vi "Flatten Readable.vi"(8 "error in (no error)":errorcluster, 11 "Reader.lvclass":refnum<class "Reader.lvclass">) -> (0 "error out":errorcluster)   [LabVIEW 2009, in "Reader.lvclass"]
uses:
  Reader.lvclass
  Reader.lvclass/Reader.ctl
  Instruments/Utility Classes/Readable/Readable.lvclass
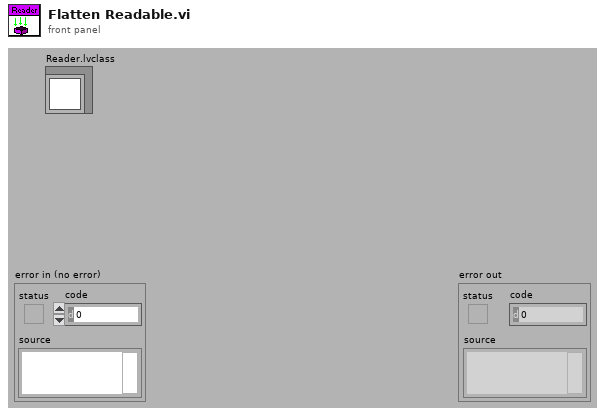
[diagram p1: front panel]
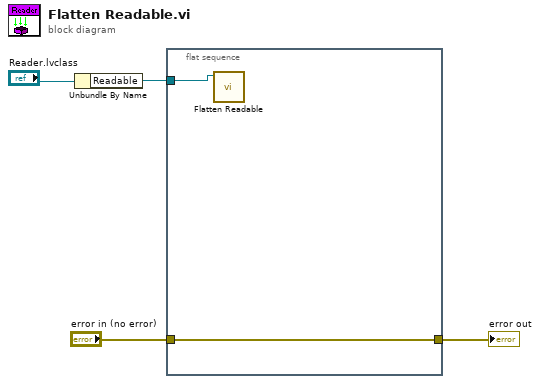
[diagram p0: block diagram]
diagram:
  n1 = Unbundle By Name("Reader.lvclass") -> ("Readable"=w3:refnum<class "Readable.lvclass">)
  n2 = flat-sequence {
    tunnel: w3 -> [w6]
    tunnel: [w5] -> w2
    tunnel: "error in (no error)" -> [w5]
    frame #0 {
      n3 = call "Flatten Readable.vi"("Readable.lvclass"=w6) -> ()  [unwired: 11 in]
    }
  }
  "error out" <- w2
